vi "NT_Cast Var Number to Dbl.vi"(8 "error in (no error)":errorcluster, 11 "NewVal":variant) -> (0 "error out":errorcluster, 2 "Numeric":dbl)   [LabVIEW 2025]
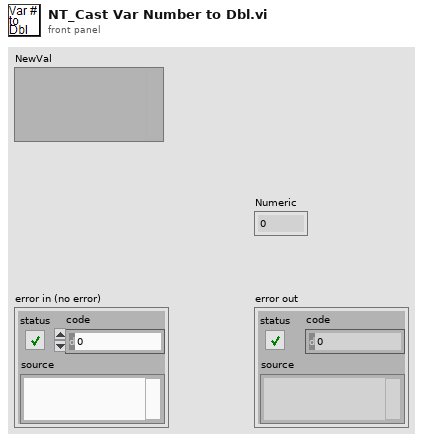
[diagram p1: front panel]
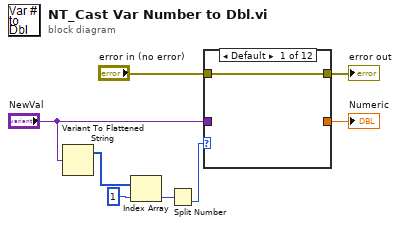
[diagram p0: block diagram]
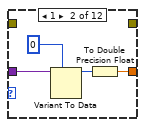
[diagram p2: hidden frame]
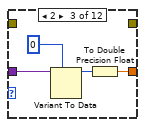
[diagram p3: hidden frame]
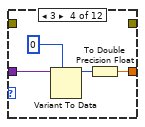
[diagram p4: hidden frame]
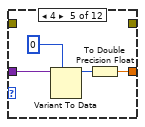
[diagram p5: hidden frame]
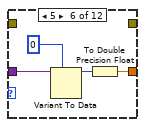
[diagram p6: hidden frame]
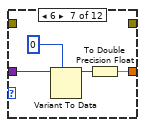
[diagram p7: hidden frame]
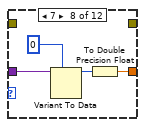
[diagram p8: hidden frame]
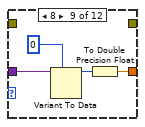
[diagram p9: hidden frame]
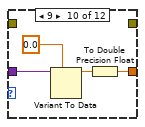
[diagram p10: hidden frame]
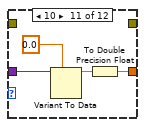
[diagram p11: hidden frame]
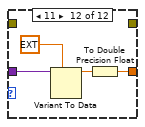
[diagram p12: hidden frame]
diagram:
  n1 = Variant To Flattened String(Variant="NewVal") -> (1:w6:i16[])  [unwired: 1 out]
  n2 = Index Array(array=w6, index=1) -> (element=w7:i16)
  n3 = Split Number(x=w7) -> (lo(x)=w8:u8)  [unwired: 1 out]
  n4 = case shown="Default" w8 {
    tunnel: "NewVal" -> [_ w13 w17 w21 w25 w29 w33 w37 w41 w45 w49 w53]
    tunnel: [_ w10 w14 w18 w22 w26 w30 w34 w38 w42 w46 w50] -> w3
    tunnel: [w9 _ _ _ _ _ _ _ _ _ _ _] -> w4
    tunnel: "error in (no error)" -> [w9 _ _ _ _ _ _ _ _ _ _ _]
    frame Default {
    }
    frame 1 {
      n5 = Variant To Data(type=i8 0, Variant=w13) -> (data=w11:i8)  [unwired: 1 in, 1 out]
      n6 = To Double Precision Float(number=w11) -> (double precision float=w10:dbl)
    }
    frame 2 {
      n7 = Variant To Data(type=i16 0, Variant=w17) -> (data=w15:i16)  [unwired: 1 in, 1 out]
      n8 = To Double Precision Float(number=w15) -> (double precision float=w14:dbl)
    }
    frame 3 {
      n9 = Variant To Data(type=0, Variant=w21) -> (data=w19:i32)  [unwired: 1 in, 1 out]
      n10 = To Double Precision Float(number=w19) -> (double precision float=w18:dbl)
    }
    frame 4 {
      n11 = Variant To Data(type=i64 0, Variant=w25) -> (data=w23:i64)  [unwired: 1 in, 1 out]
      n12 = To Double Precision Float(number=w23) -> (double precision float=w22:dbl)
    }
    frame 5 {
      n13 = Variant To Data(type=u8 0, Variant=w29) -> (data=w27:u8)  [unwired: 1 in, 1 out]
      n14 = To Double Precision Float(number=w27) -> (double precision float=w26:dbl)
    }
    frame 6 {
      n15 = Variant To Data(type=u16 0, Variant=w33) -> (data=w31:u16)  [unwired: 1 in, 1 out]
      n16 = To Double Precision Float(number=w31) -> (double precision float=w30:dbl)
    }
    frame 7 {
      n17 = Variant To Data(type=u32 0, Variant=w37) -> (data=w35:u32)  [unwired: 1 in, 1 out]
      n18 = To Double Precision Float(number=w35) -> (double precision float=w34:dbl)
    }
    frame 8 {
      n19 = Variant To Data(type=u64 0, Variant=w41) -> (data=w39:u64)  [unwired: 1 in, 1 out]
      n20 = To Double Precision Float(number=w39) -> (double precision float=w38:dbl)
    }
    frame 9 {
      n21 = Variant To Data(type=sgl 0.0, Variant=w45) -> (data=w43:sgl)  [unwired: 1 in, 1 out]
      n22 = To Double Precision Float(number=w43) -> (double precision float=w42:dbl)
    }
    frame 10 {
      n23 = Variant To Data(type=0.0, Variant=w49) -> (data=w47:dbl)  [unwired: 1 in, 1 out]
      n24 = To Double Precision Float(number=w47) -> (double precision float=w46:dbl)
    }
    frame 11 {
      n25 = Variant To Data(type=ext 0.0, Variant=w53) -> (data=w51:ext)  [unwired: 1 in, 1 out]
      n26 = To Double Precision Float(number=w51) -> (double precision float=w50:dbl)
    }
  }
  "error out" <- w4
  "Numeric" <- w3
